vi "GV preline.vi"() -> ()   [LabVIEW 2017]
panel:
  out "Preline":bool
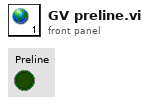
[diagram p1: front panel]
diagram:
